vi "index power set-get all subsets of specified length.vi"(8 "error in (no error)":errorcluster, 10 "Desired subsets length":i32=3, 11 "End index":i32=5) -> (0 "error out":errorcluster, 2 "no. of subsets":i32, 3 "Subsets of indexes":variant[](array[variant]))   [LabVIEW 2021, in "Numeric Utilities.lvlib"]
uses:
  Numeric Utilities.lvlib
  cluster-touched index.ctl
  index state enum.ctl
panel:
  in  "Dev: Stop Button":bool
  out "Pool":T1[](array[typedef])
  out "Loop iteration":i32
  out "State transition":string[](array[string])
  out "T = there are enough elements to the right of \"current index\" to form at least one subset of the desired length":bool
  # "Development\ncontrols/indicators useful for development and testing, but which are not outputs of the VI"
  # "Input\nInputs to the VI"
  # "Output\nOutputs of the VI"
  # "Description\n\nBlank VI with error handling case. \n\nSummarize the use of this VI in this space."
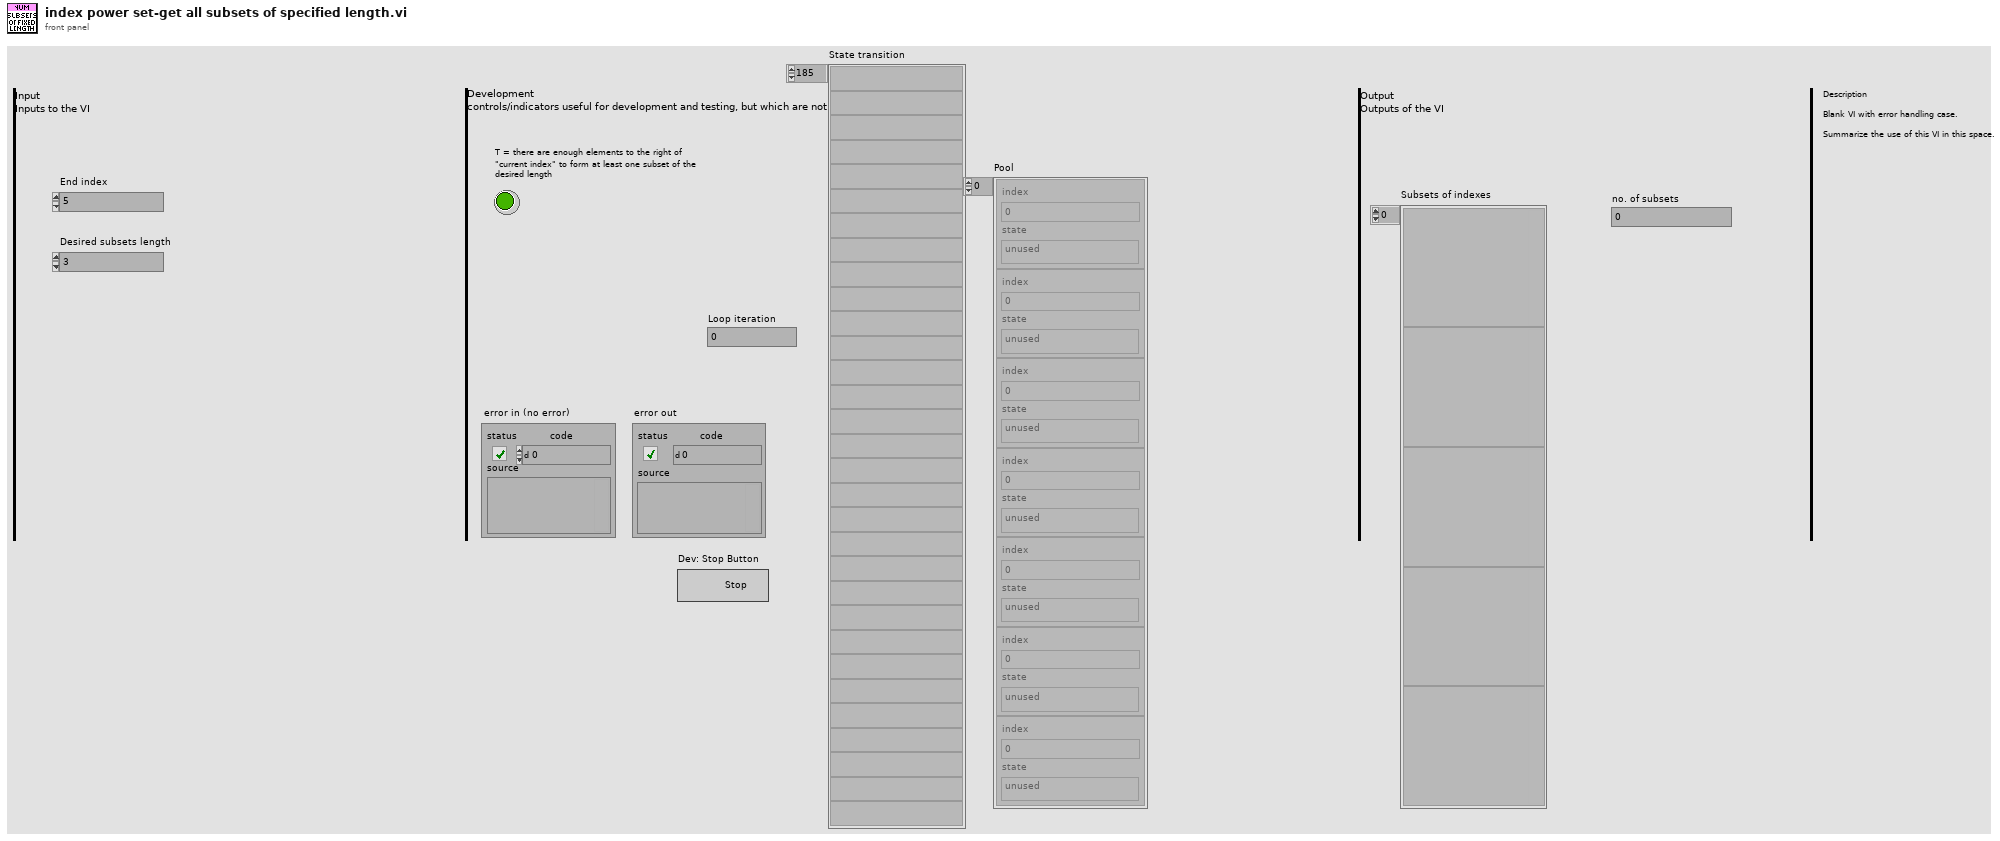
[diagram p1: front panel]
types:
  T1 = typedef "Numeric Utilities.lvlib/cluster-touched index.ctl" = cluster{"index":i32, "state":T2}
  T2 = typedef "Numeric Utilities.lvlib/index state enum.ctl" = enum16{"unused", "selected", "exhausted"}
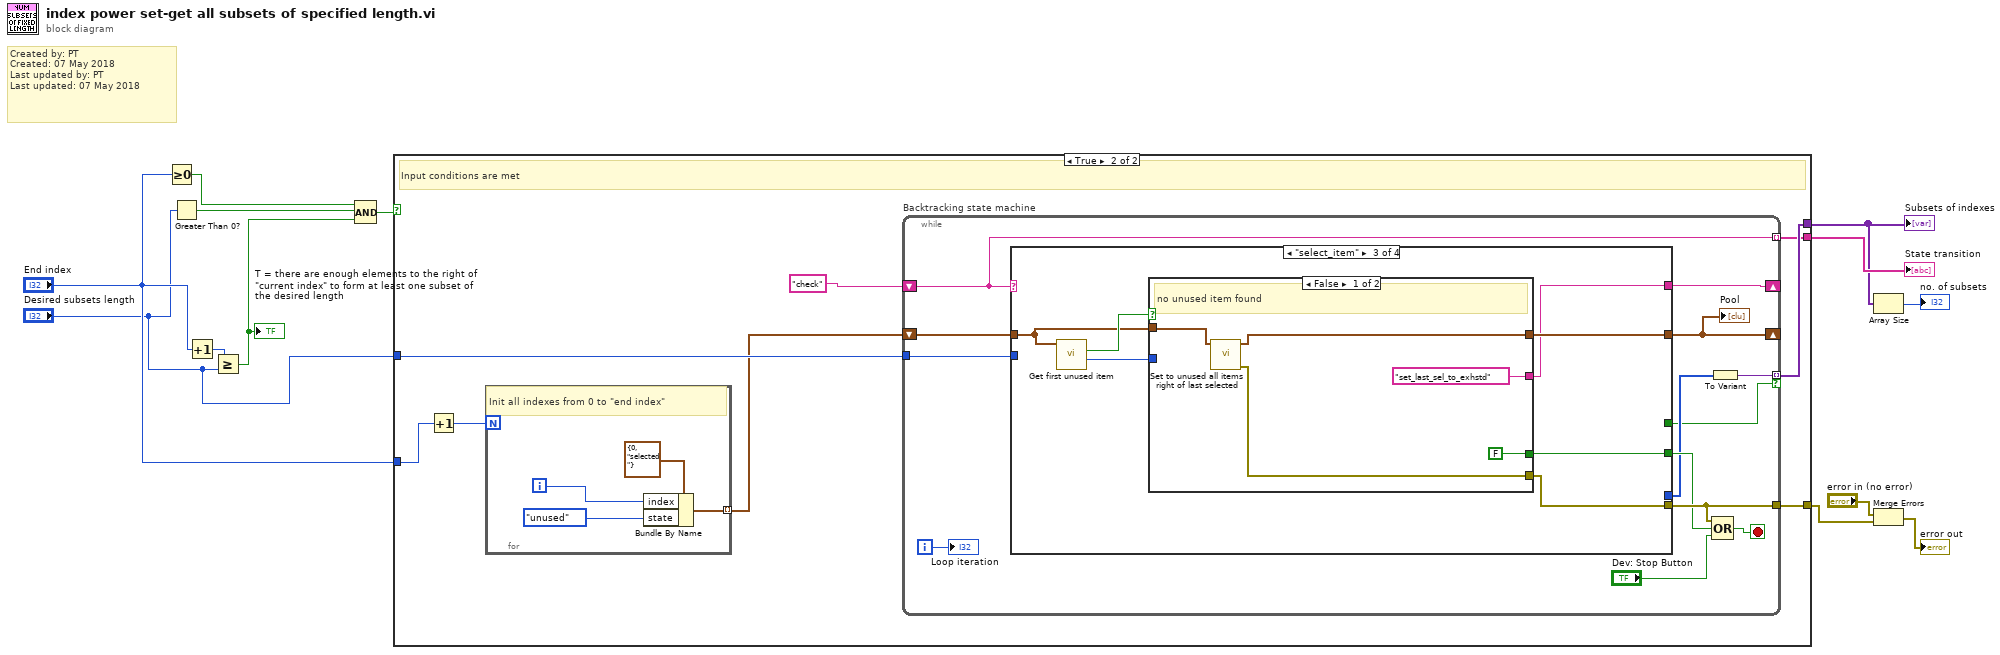
[diagram p0: block diagram]
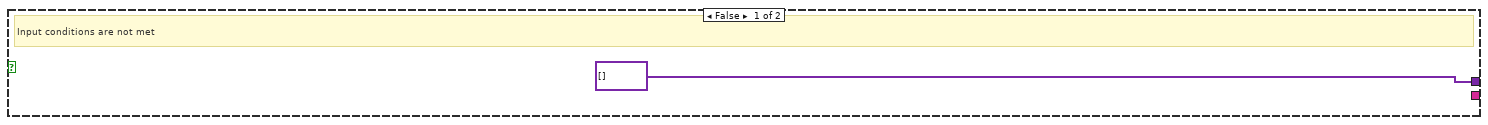
[diagram p2: hidden frame]
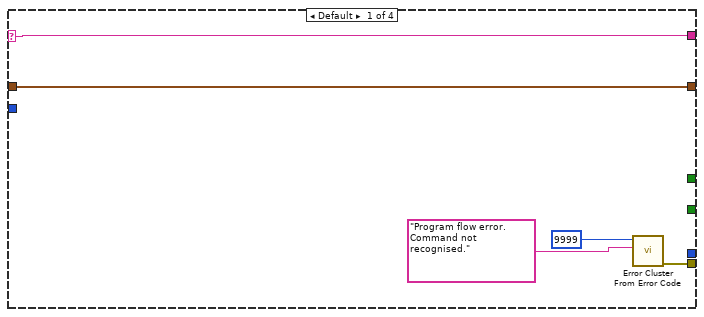
[diagram p3: hidden frame]
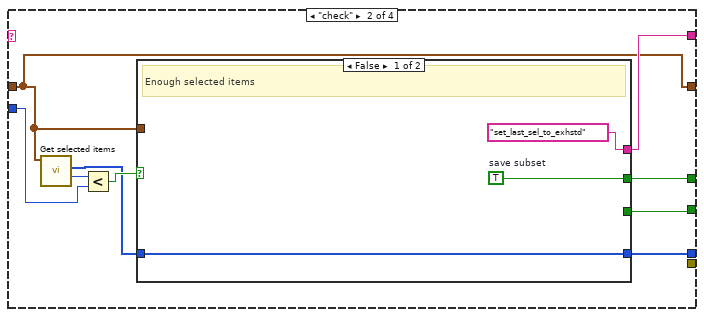
[diagram p4: hidden frame]
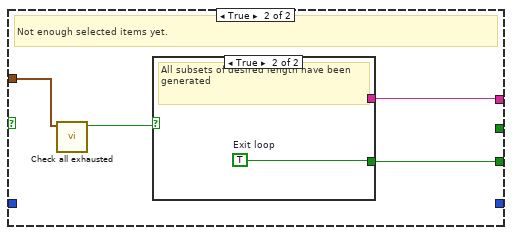
[diagram p5: hidden frame]
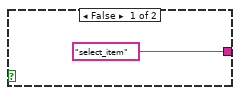
[diagram p6: hidden frame]
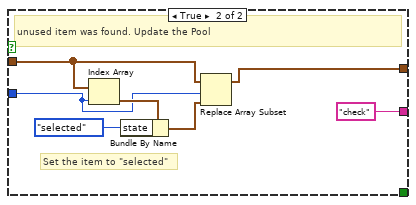
[diagram p7: hidden frame]
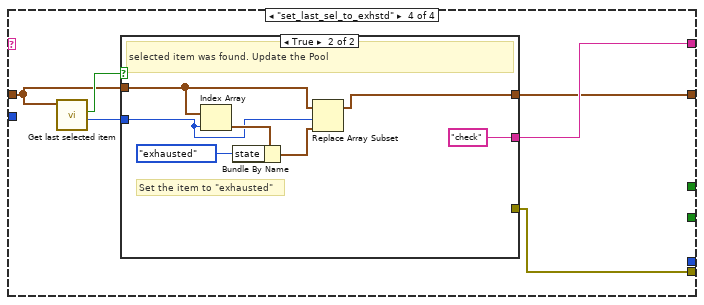
[diagram p8: hidden frame]
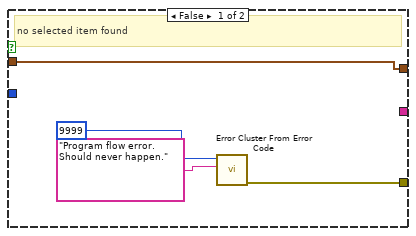
[diagram p9: hidden frame]
diagram:
  # "Created by: PT\nCreated: 07 May 2018\nLast updated by: PT\nLast updated: 07 May 2018"
  n1 = Greater Or Equal To 0?(x="End index") -> (x >= 0?=w13:bool)
  n2 = Greater Than 0?(x="Desired subsets length") -> (x > 0?=w12:bool)
  n3 = Increment(x="End index") -> (x+1=w10:i32)
  n4 = Greater Or Equal?(x=w10, y="Desired subsets length") -> (x >= y?=w1:bool)
  "T = there are enough elements to the right of \"current index\" to form at least one subset of the desired length" <- w1
  n5 = Compound Arithmetic op=AND(w13, w12, w1) -> (w5:bool)
  n6 = case shown="True" w5 {
    tunnel: [variant[] [] ("Subsets of indexes") w16] -> w3
    tunnel: "Desired subsets length" -> [_ w21]
    tunnel: "End index" -> [_ w20]
    tunnel: [_ w17] -> w7
    tunnel: [_ w15] -> w4
    frame False {
      # "Input conditions are not met"
    }
    frame True {
      # "Input conditions are met"
      n7 = Increment(x=w20) -> (x+1=w19:i32)
      n8 = for {
        N: w19 -> [_]
        tunnel: [w23] -> w18 mode=indexing
        i -> [w25]
        # "Init all indexes from 0 to \"end index\""
        n9 = Bundle By Name(cluster=T1 {"index"=0, "state"=enum."selected"} ("index"), "index"=w25, "state"=index_state_enum."unused" ("touched enum")) -> (w23:T1)
      }
      n10 = while "Backtracking state machine" {
        tunnel: w21 -> [w39]
        shift-right: [w38] -> _
        shift-left: "check" -> [w29]
        shift-right: [w36] -> _
        shift-left: w18 -> [w37]
        tunnel: [w34] -> w17
        tunnel: [w31] -> w16 mode=indexing if=w30
        tunnel: [w29] -> w15 mode=indexing
        i -> [w28]
        stop <- w35 stop-if-true
        n11 = case shown="\"select_item\"" w29 {
          selector: w29 -> [w40 _ _ _]
          tunnel: w39 -> [_ w52 _ _]
          tunnel: [w40 w50 w64 w84] -> w38
          tunnel: w37 -> [w44 w48 w68 w86]
          tunnel: [w44 w48 w66 w83] -> w36
          tunnel: [w41 _ w63 w82] -> w34
          tunnel: [_ w47 w65 _] -> w33
          tunnel: [_ w45 _ _] -> w32
          tunnel: [_ w49 _ _] -> w30
          frame Default {
            n12 = call <vilib>:"Error Cluster From Error Code.vi"("error message (\"\")"="Program flow error. Command not recognised.", "error code (0)"=9999) -> ("error out"=w41:errorcluster)  [unwired: 7 in]
          }
          frame "check" {
            n13 = call "Get selected items.vi"("Pool"=w48) -> ("no. of selected items"=w53:i32, "Selected indexes"=w46:i32[])  [unwired: 7 in, 2 out]
            n14 = Less?(x=w53, y=w52) -> (x < y?=w51:bool)
            n15 = case shown="False" w51 {
              tunnel: ["set_last_sel_to_exhstd" w60] -> w50
              tunnel: [w56 _] -> w49
              tunnel: w48 -> [_ w59]
              tunnel: [_ w57] -> w47
              tunnel: w46 -> [w54 _]
              tunnel: [w54 _] -> w45
              frame False {
                w56 = TRUE  # save subset
                # "Enough selected items"
              }
              frame True {
                # "Not enough selected items yet."
                n16 = call "Check all exhausted.vi"("Pool"=w59) -> ("T = all items are \"exhausted\""=w58:bool)  [unwired: 9 in, 1 out]
                n17 = case shown="True" w58 {
                  tunnel: ["select_item" _] -> w60
                  tunnel: [_ w62] -> w57
                  frame False {
                  }
                  frame True {
                    w62 = TRUE  # Exit loop
                    # "All subsets of desired length have been generated"
                  }
                }
              }
            }
          }
          frame "select_item" {
            n18 = call "Get first unused item.vi"("Pool"=w68) -> ("index of first unused item"=w67:i32, "T = unused item was found"=w69:bool)  [unwired: 7 in, 2 out]
            n19 = case shown="False" w69 {
              tunnel: w68 -> [w72 w81]
              tunnel: w67 -> [_ w77]
              tunnel: [w71 w76] -> w66
              tunnel: [FALSE _] -> w65
              tunnel: ["set_last_sel_to_exhstd" "check"] -> w64
              tunnel: [w70 _] -> w63
              frame False {
                # "no unused item found"
                n20 = call "Set to unused all items right of last selected.vi"("Pool in"=w72) -> ("error out"=w70:errorcluster, "Pool out"=w71:T1[])  [unwired: 9 in]
              }
              frame True {
                # "Set the item to \"selected\""
                # "unused item was found. Update the Pool"
                n21 = Index Array(array=w81, index=w77) -> (element=w80:T1)
                n22 = Bundle By Name(cluster=w80, "state"=index_state_enum."selected") -> (w78:T1)
                n23 = Replace Array Subset(array=w81, new element=w78, index=w77) -> (w76:T1[])
              }
            }
          }
          frame "set_last_sel_to_exhstd" {
            n24 = call "Get last selected item.vi"("Pool"=w86) -> ("index of last selected item"=w85:i32, "T = selected item was found"=w87:bool)  [unwired: 7 in, 2 out]
            n25 = case shown="True" w87 {
              tunnel: w86 -> [w91 w98]
              tunnel: w85 -> [_ w94]
              tunnel: [w91 w93] -> w83
              tunnel: [_ "check"] -> w84
              tunnel: [w88 _] -> w82
              frame False {
                # "no selected item found"
                n26 = call <vilib>:"Error Cluster From Error Code.vi"("error message (\"\")"="Program flow error. Should never happen.", "error code (0)"=9999) -> ("error out"=w88:errorcluster)  [unwired: 7 in]
              }
              frame True {
                # "Set the item to \"exhausted\""
                # "selected item was found. Update the Pool"
                n27 = Index Array(array=w98, index=w94) -> (element=w97:T1)
                n28 = Bundle By Name(cluster=w97, "state"=index_state_enum."exhausted") -> (w95:T1)
                n29 = Replace Array Subset(array=w98, new element=w95, index=w94) -> (w93:T1[])
              }
            }
          }
        }
        "Pool" <- w36
        n30 = To Variant(anything=w32) -> (Variant=w31:variant)
        n31 = Compound Arithmetic op=OR(w34, w33, "Dev: Stop Button") -> (w35:bool)
        "Loop iteration" <- w28
      }
    }
  }
  "Subsets of indexes" <- w3
  "State transition" <- w4
  n32 = Array Size(array=w3) -> (size(s)=→"no. of subsets":i32)
  n33 = Merge Errors("error in (no error)", w7) -> (→"error out":errorcluster)
